vi "ScopeTest.vi"() -> ()   [LabVIEW 2018]
uses:
  <vilib>/measure/mascope.llb/Pulse Measurements 1 chan.vi
  <instrlib>/RIGOL DS1000 Series/RIGOL DS1000 Series.lvlib
  <vilib>/measure/NI_MAPro.lvlib
panel:
  out "x/y":dbl
  out "period":dbl format="%.2g"
  in  "VISA resource name 2":refnum<visa-resource-name>="USB0::0x1AB1::0x0641::DG4E202501630::INSTR"
  in  "VISA resource name":refnum<visa-resource-name>="DemoScope"
  out "Waveform Data":waveform(dbl)(graph)
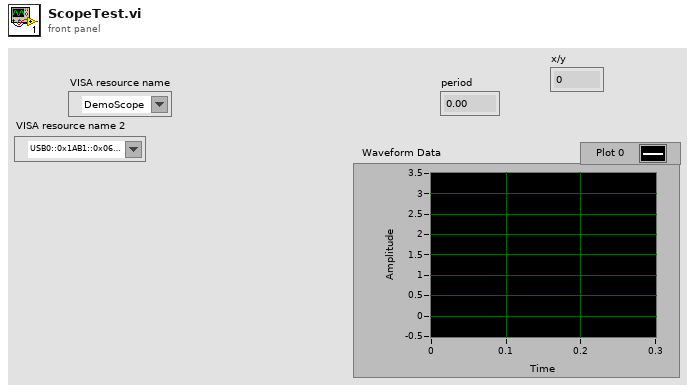
[diagram p1: front panel]
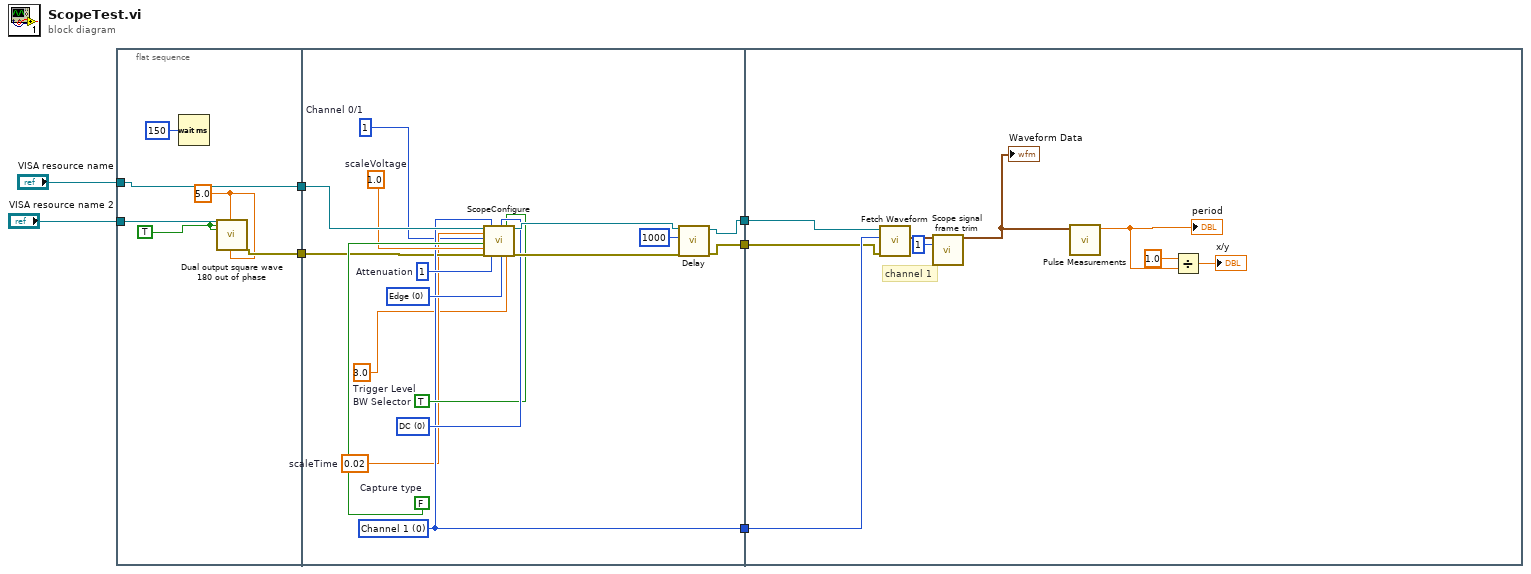
[diagram p0: block diagram]
diagram:
  n1 = flat-sequence {
    tunnel: "VISA resource name" -> [w9]
    tunnel: [w13] -> w6
    tunnel: "VISA resource name 2" -> [w12]
    tunnel: [w9] -> w3
    tunnel: [w21] -> w4
    tunnel: w6 -> [w20]
    tunnel: w3 -> [w30]
    tunnel: [w15] -> w2
    tunnel: [w14] -> w1
    tunnel: w4 -> [w39]
    tunnel: w2 -> [w37]
    tunnel: w1 -> [w36]
    frame #0 {
      w8 = 5.0 ("Frequency 1")
      w10 = TRUE ("Enable Output 1")
      n2 = Wait (ms)(milliseconds to wait=u32 150) -> ()  [unwired: 1 out]
      n3 = call "Dual output square wave 180 out of phase.vi"("VISA resource name"=w12, "Enable Output 1"=w10, "Enable Align (F: Disable) 1"=w10, "Frequency 1"=w8, "Frequency 2"=w8) -> ("error out"=w13:errorcluster)  [unwired: 21 in, 1 out]
    }
    frame #1 {
      w17 = 1  # Channel 0/1
      w27 = FALSE  # Capture type
      w22 = u16 0 items=["Edge", "Pulse", "Video", "Pattern", "Duration"] ("Trigger Type (0: Edge)")
      w18 = 3.0  # Trigger Level
      w25 = u16 0 items=["DC", "AC", "Ground"] ("Vertical Coupling (0: DC)")
      w23 = 1  # Attenuation
      w26 = 1.0  # scaleVoltage
      w19 = 0.02  # scaleTime
      w24 = TRUE  # BW Selector
      w21 = u16 0 items=["Channel 1", "Channel 2", "Channel 3", "Channel 4"] ("Channel (0: Channel 1)")
      n4 = call "ScopeConfigure.vi"("VISA resource name"=w30, "scaleTime"=w19, "Channel 0/1"=w17, "Single Capture"=w27, "scaleVoltage"=w26, "error in (no error)"=w20, "Channel (0: Channel 1)"=w21, "Attenuation"=w23, "Vertical Coupling (0: DC)"=w25, "Trigger Type (0: Edge)"=w22, "BW Selector"=w24, "Trigger Level"=w18) -> ("VISA resource name out"=w29:refnum<visa-resource-name>, "error out"=w28:errorcluster)  [unwired: 6 in]
      n5 = call <instrlib>:"Delay.vi"("error in (no error)"=w28, "Delay (ms)"=u32 1000, "VISA resource name"=w29) -> ("error out"=w15:errorcluster, "VISA resource name out"=w14:refnum<visa-resource-name>)  [unwired: 7 in]
    }
    frame #2 {
      # "channel 1"
      n6 = call <instrlib>:"Fetch Waveform.vi"("error in (no error)"=w37, "Channel (0: Channel 1)"=w39, "VISA resource name"=w36) -> ("Waveform Data"=w38:waveform(dbl))  [unwired: 6 in, 2 out]
      n7 = call "Scope signal frame trim.vi"("Waveform Data"=w38, "Frame delete"=1) -> ("waveform out"=w32:waveform(dbl))  [unwired: 12 in, 1 out]
      "Waveform Data" <- w32
      n8 = call-poly <vilib>:"Pulse Measurements.vi"("signal in"=w32) -> ("period"=w35:dbl)  [unwired: 6 in, 4 out]
      "period" <- w35
      n9 = Divide(x=1.0, y=w35) -> (x/y=→"x/y":dbl)
    }
  }
